vi "Triangle Begin.vi"   [LabVIEW 2012]
uses:
  <vilib>/Rock Robotics/SystemInterfaces/Typedef/FPGA_TypedefDigitalModule.ctl
  <vilib>/Rock Robotics/SystemInterfaces/DIO/FPGA_DIOPWMChannel.ctl
  <vilib>/Rock Robotics/WPI/MotorControl/WPI_MotorControlOpen Jaguar.vi
types:
  T1 = typedef "FPGA_DIOPWMChannel.ctl" = enum8{"PWM 1", "PWM 2", "PWM 3", "PWM 4", "PWM 5", "PWM 6", "PWM 7", "PWM 8", "PWM 9", "PWM 10", "Invalid"}
  T2 = typedef "FPGA_TypedefDigitalModule.ctl" = enum16{"Digital Module 1", "Digital Module 2"}
  T3 = typedef "WPI_MotorControlDeviceRef.ctl" = cluster{"DeviceStatus":errorcluster, "Type":enum16{"PWM", "CAN"}, "PWM":cluster{"Digital Module":T2, "PWM Channel":T1, "DeadBand":T4}, "CAN":cluster{"Device Number":u8, "Control Mode":T5, "Semaphore":T6, "Max Vout":dbl}, "Invert":bool, "TransformRef":T7, "InvTransformRef":T7}
  T4 = typedef "WPI_PWMDeadband.ctl" = cluster{"Name":string, "maxPositivePwm":i32, "minPositivePwm":i32, "centerPwm":i32, "maxNegativePwm":i32, "minNegativePwm":i32, "angularRange":u16}
  T5 = typedef "WPI_CANJaguar_ControlMode.ctl" = enum8{"Percent VBus", "Current", "Speed", "Position", "Voltage"}
  T6 = typedef "Semaphore RefNum" = refnum<k1>
  T7 = typedef "WPI_PWMTransform_ConPane.ctl" = refnum<vi>
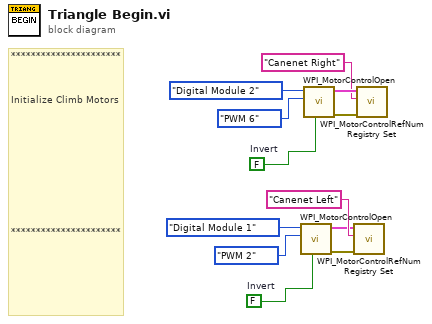
[diagram p0: block diagram]
diagram:
  w5 = FALSE  # Invert
  w8 = FALSE  # Invert
  # "**********************\n\n\n\nInitialize Climb Motors          \n\n\n\n\n\n\n\n\n\n\n\n**********************"
  n1 = call-poly <vilib>:"WPI_MotorControlOpen.vi"("Invert"=w5, "PWM Channel"=FPGA_DIOPWMChannel."PWM 2", "Digital Module (Module 1)"=FPGA_TypedefDigitalModule."Digital Module 1") -> ("error out"=w6:errorcluster, "MotorControlDeviceRef"=w1:T3)  [unwired: 7 in]
  n2 = call-poly <vilib>:"WPI_MotorControlOpen.vi"("Invert"=w8, "PWM Channel"=FPGA_DIOPWMChannel."PWM 6", "Digital Module (Module 1)"=FPGA_TypedefDigitalModule."Digital Module 2") -> ("error out"=w7:errorcluster, "MotorControlDeviceRef"=w12:T3)  [unwired: 7 in]
  n3 = call <vilib>:"WPI_MotorControlRefNum Registry Set.vi"("error in (no error)"=w6, "refnum name"="Canenet Left", "MotorControlDevRef"=w1) -> ()  [unwired: 7 in, 2 out]
  n4 = call <vilib>:"WPI_MotorControlRefNum Registry Set.vi"("error in (no error)"=w7, "refnum name"="Canenet Right", "MotorControlDevRef"=w12) -> ()  [unwired: 7 in, 2 out]
